vi "EX_OUT_On_Off.vi"(8 "错误输入（无错误）":errorcluster, 10 "Mode":enum16{"ON", "OFF"}(ring), 11 "VISA resource name":refnum<visa-resource-name> caption="VISA资源名称") -> (0 "error out":errorcluster caption="错误输出", 3 "VISA资源名称输出":refnum<visa-resource-name>)   [LabVIEW 2017]
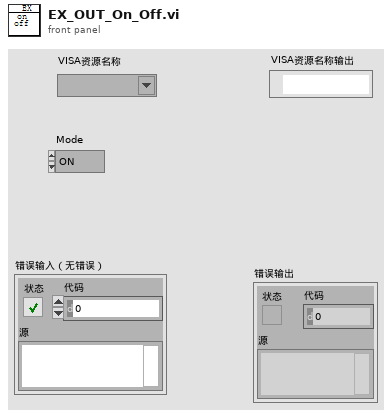
[diagram p1: front panel]
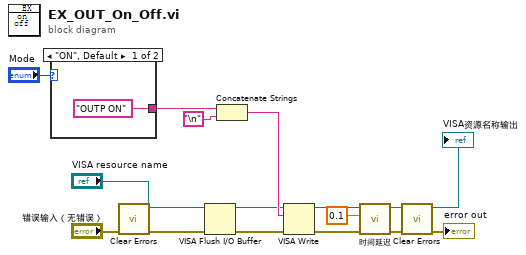
[diagram p0: block diagram]
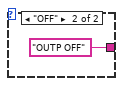
[diagram p2: hidden frame]
diagram:
  n1 = case shown="\"ON\", Default" "Mode" {
    tunnel: ["OUTP ON" "OUTP OFF"] -> w10
    frame "ON", Default {
    }
    frame "OFF" {
    }
  }
  n2 = call <vilib>:"Clear Errors.vi"("error in (no error)"="错误输入（无错误）") -> ("error out"=w1:errorcluster)  [unwired: 5 in, 1 out]
  n3 = VISA Flush I/O Buffer(VISA resource name="VISA resource name", error in (no error)=w1) -> (VISA resource name out=w4:refnum<visa-resource-name>, error out=w2:errorcluster)  [unwired: 1 in]
  n4 = Concatenate Strings(w10, "\n") -> (w11:string)
  n5 = VISA Write(VISA resource name=w4, write buffer=w11, error in (no error)=w2) -> (VISA resource name out=→"VISA资源名称输出":refnum<visa-resource-name>, error out=w14:errorcluster)  [unwired: 1 out]
  n6 = call "时间延迟"("error in (no error)"=w14, "Delay Time (s)"=0.1) -> ("error out"=w8:errorcluster)  [unwired: 9 in]
  n7 = call <vilib>:"Clear Errors.vi"("error in (no error)"=w8) -> ("error out"=→"error out":errorcluster)  [unwired: 5 in, 1 out]
